vi "Test Class.vi"() -> ()   [LabVIEW 2013]
uses:
  <vilib>/Utility/miscctls.llb/LVRGBAColorTypeDef.ctl
  Trajectory Drawer.lvclass
  <vilib>/Platform/TimedLoop/XDataNode/timing_clust.ctl
  <vilib>/Platform/TimedLoop/XDataNode/nitl_modes.ctl
  <vilib>/Platform/TimedLoop/XDataNode/wakeup.ctl
  <vilib>/picture/3D Picture Control/Object/Create Object (name).vi
  <vilib>/platform/TimedLoop/XDataNode/XDataNode.xnode
  <vilib>/Platform/TimedLoop/XDataNode/XDNodeRunTimeDep.lvlib
  <vilib>/picture/3D Picture Control/NI_3D Picture Control.lvlib
panel:
  in  "stop 2":bool
  in  "stop":bool
  out "3D Picture":refnum<vi>(3d-picture)
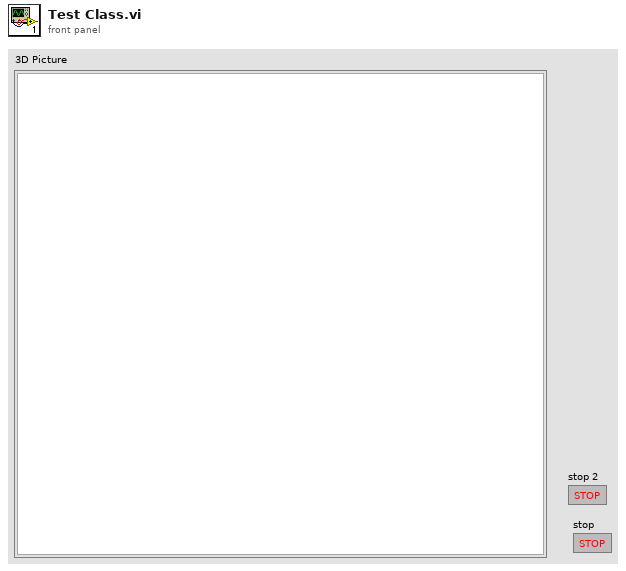
[diagram p1: front panel]
types:
  T1 = typedef "LVRGBAColorTypeDef.ctl" = cluster{"Red":sgl, "Green":sgl, "Blue":sgl, "Alpha":sgl}
  T2 = enum16{"Inherit Value", "Points", "Wireframe", "Polygons"}
  T3 = typedef "XDNodeRunTimeDep.lvlib/timing_clust.ctl" = cluster{"Expected End [f-1]":u64, "Actual End [f-1]":u64, "Finished Late? [f-1]":bool, "Expected End [i-1]":u64, "Actual End [i-1]":u64, "Finished Late? [i-1]":bool, "Expected Start [i]":u64, "Actual Start [i]":u64, "Expected Start [f]":u64, "Actual Start [f]":u64, "Source Name":string, "Structure Name":string, "Period":i64, "Deadline":i64, "Offset":i64, "Start":i64, "Priority":i32, "Timeout":i32, "Mode":T4, "Wakeup Reason":T5, "Error":errorcluster, "Source Type":string, "Secondary Source Type":string, "Global End Time":u64, "Global Start Time":u64, "Frame Duration":u64, "Iteration Duration":u64, "Assigned CPU":i32, "I/O Scan Engine Mode":u32}
  T4 = typedef "XDNodeRunTimeDep.lvlib/nitl_modes.ctl" = enum32{"No Change", "Process missed periods, maintain original phase", "Discard missed periods, maintain original phase", "Process missed periods, ignore original phase", "Discard missed periods, ignore original phase"}
  T5 = typedef "XDNodeRunTimeDep.lvlib/wakeup.ctl" = enum32{"Normal", "Aborted", "Asynchronous wakeup", "Timing source error", "Timed loop error", "Timeout"}
  T6 = cluster{"number: 0 to 1":dbl, "number: 0 to 1":dbl, "number: 0 to 1":dbl}
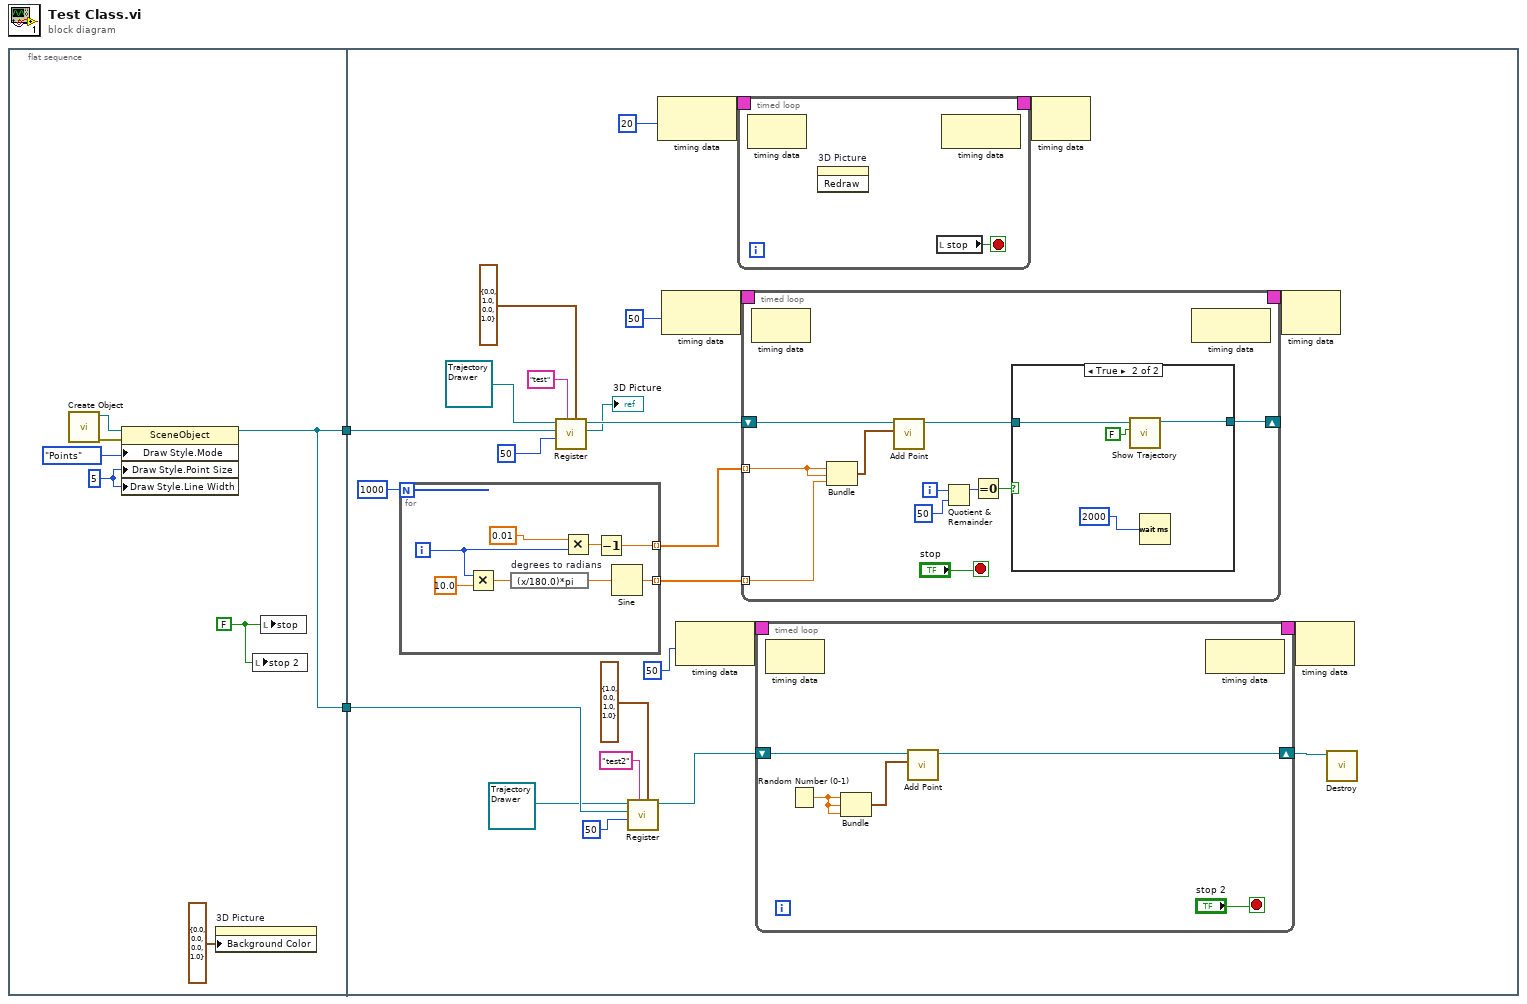
[diagram p0: block diagram]
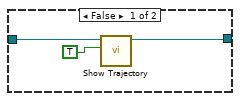
[diagram p2: hidden frame]
diagram:
  n1 = flat-sequence {
    tunnel: [w5] -> w2
    tunnel: [w5] -> w1
    tunnel: w2 -> [w22]
    tunnel: w1 -> [w20]
    frame #0 {
      w7 = 5
      w4 = FALSE
      n2 = call-poly <vilib>:"Create Object.vi"() -> ("error out"=w6:errorcluster, "Scene:New Object"=w9:refnum<vi>)  [unwired: 10 in]
      n3 = property class="SceneObject"(reference=w9, error in=w6, "Draw Style.Mode"=T2."Points" ("Draw Style:Mode"), "Draw Style.Point Size"=w7, "Draw Style.Line Width"=w7) -> (reference out=w5:refnum<vi>)  [unwired: 1 out]
      n4 = property on="3D Picture" class="SceneGraphDisp (strict)"("Background Color"=T1 {"Red"=0.0, "Green"=0.0, "Blue"=0.0, "Alpha"=1.0}) -> ()  [unwired: 2 in, 2 out]
      n5 = local write "stop 2"(w4) -> ()
      n6 = local write "stop"(w4) -> ()
    }
    frame #1 {
      n7 = for {
        N: 1000 -> [_]
        tunnel: [w59] -> w29 mode=indexing
        tunnel: [w54] -> w16 mode=indexing
        i -> [w58]
        n8 = Multiply(x=w58, y=10.0) -> (x*y=w56:dbl)
        n9 = expression code="(x/180.0)*pi" "degrees to radians"(w56) -> (w55:dbl)
        n10 = Multiply(x=0.01, y=w58) -> (x*y=w60:dbl)
        n11 = Decrement(x=w60) -> (x-1=w59:dbl)
        n12 = Sine(x=w55) -> (sin(x)=w54:dbl)
      }
      n13 = call-dynamic "Register.vi"("Color"=T1 {"Red"=0.0, "Green"=1.0, "Blue"=0.0, "Alpha"=1.0}, "Name"="test", "Capacity"=50, "Root Sence"=w22, "Trace Drawer in"=refnum<class "Trajectory Drawer.lvclass"> refnum ("Trace Drawer.lvclass")) -> ("Root Sence Out"=→"3D Picture":refnum<vi>, "Trace Drawer out"=w26:refnum<class "Trajectory Drawer.lvclass">)  [unwired: 4 in, 1 out]
      n14 = call-dynamic "Register.vi"("Color"=T1 {"Red"=1.0, "Green"=0.0, "Blue"=1.0, "Alpha"=1.0}, "Name"="test2", "Capacity"=50, "Root Sence"=w20, "Trace Drawer in"=refnum<class "Trajectory Drawer.lvclass"> refnum ("Trajectory Drawer.lvclass")) -> ("Trace Drawer out"=w15:refnum<class "Trajectory Drawer.lvclass">)  [unwired: 4 in, 2 out]
      n15 = node-c288(20) -> (w33:T3)
      n16 = node-c288(50) -> (w35:T3)
      n17 = node-c288(50) -> (w18:T3)
      n18 = timed-loop {
        timing: w33 -> [_]
        timing-out: [_] -> w32
        stop <- w47 stop-if-true
        n19 = node-c288() -> ()  [unwired: 1 in, 1 out]
        n20 = invoke on="3D Picture" class="SceneGraphDisp (strict)" method="Redraw"() -> ()  [unwired: 3 in, 3 out]
        n21 = local read "stop"() -> (w47:bool)
        n22 = node-c288() -> ()  [unwired: 1 in, 1 out]
      }
      n23 = timed-loop {
        timing: w35 -> [_]
        timing-out: [_] -> w34
        shift-right: [w62] -> _
        shift-left: w26 -> [w69]
        tunnel: w29 -> [w72] mode=indexing
        tunnel: w16 -> [w70] mode=indexing
        i -> [w67]
        stop <- "stop" stop-if-true
        n24 = node-c288() -> ()  [unwired: 1 in, 1 out]
        n25 = Bundle(w72, w72, w70) -> (w68:cluster{dbl, dbl, dbl})  [unwired: 1 in]
        n26 = call-dynamic "Add Point.vi"("3D Point"=w68, "Trajectory Drawer in"=w69) -> ("Trajectory Drawer out"=w63:refnum<class "Trajectory Drawer.lvclass">)  [unwired: 8 in, 1 out]
        n27 = Quotient & Remainder(x=w67, y=50) -> (x-y*floor(x/y)=w65:i32)  [unwired: 1 out]
        n28 = Equal To 0?(x=w65) -> (x = 0?=w64:bool)
        n29 = case shown="True" w64 {
          tunnel: w63 -> [w75 w79]
          tunnel: [w74 w78] -> w62
          frame False {
            n30 = call-dynamic "Show Trajectory.vi"("Show?"=TRUE, "Trajectory Drawer in"=w75) -> ("Trajectory Drawer out"=w74:refnum<class "Trajectory Drawer.lvclass">)  [unwired: 8 in, 1 out]
          }
          frame True {
            n31 = call-dynamic "Show Trajectory.vi"("Show?"=FALSE, "Trajectory Drawer in"=w79) -> ("Trajectory Drawer out"=w78:refnum<class "Trajectory Drawer.lvclass">)  [unwired: 8 in, 1 out]
            n32 = Wait (ms)(milliseconds to wait=2000) -> ()  [unwired: 1 out]
          }
        }
        n33 = node-c288() -> ()  [unwired: 1 in, 1 out]
      }
      n34 = timed-loop {
        timing: w18 -> [_]
        timing-out: [_] -> w17
        shift-right: [w36] -> w13
        shift-left: w15 -> [w39]
        stop <- "stop 2" stop-if-true
        n35 = node-c288() -> ()  [unwired: 1 in, 1 out]
        n36 = Random Number (0-1)() -> (number: 0 to 1=w38:dbl)
        n37 = Bundle("number: 0 to 1"=w38, "number: 0 to 1"=w38, "number: 0 to 1"=w38) -> (w37:T6)  [unwired: 1 in]
        n38 = call-dynamic "Add Point.vi"("3D Point"=w37, "Trajectory Drawer in"=w39) -> ("Trajectory Drawer out"=w36:refnum<class "Trajectory Drawer.lvclass">)  [unwired: 8 in, 1 out]
        n39 = node-c288() -> ()  [unwired: 1 in, 1 out]
      }
      n40 = node-c288(w32) -> ()  [unwired: 1 out]
      n41 = node-c288(w34) -> ()  [unwired: 1 out]
      n42 = node-c288(w17) -> ()  [unwired: 1 out]
      n43 = call-dynamic "Destroy.vi"("Trajectory Drawer in"=w13) -> ()  [unwired: 8 in, 3 out]
    }
  }
